vi "get_component_type_name.vi"(8 "error in (no error)":errorcluster, 11 "GenericDisplay in":refnum<class "GenericDisplay.lvclass">) -> (0 "error out":errorcluster, 2 "component type":string="Display", 3 "GenericDisplay out":refnum<class "GenericDisplay.lvclass">)   [LabVIEW 2010, in "GenericDisplay.lvclass"]
uses:
  GenericDisplay.lvclass
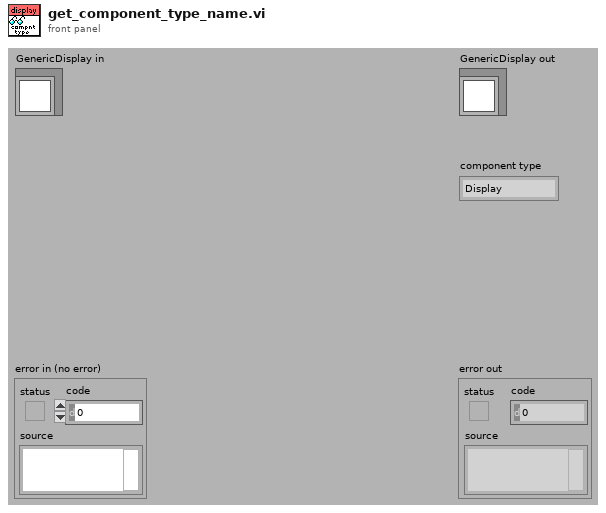
[diagram p1: front panel]
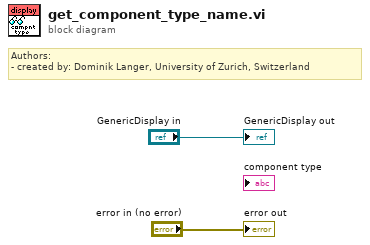
[diagram p0: block diagram]
diagram:
  # "Authors: \n- created by: Dominik Langer, University of Zurich, Switzerland"
  "error out" <- "error in (no error)"
  "GenericDisplay out" <- "GenericDisplay in"
